vi "Pulse convert.vi"(11 "PulseIN":i32) -> (2 "Speed(rpm)":i16, 3 "Speed(rad/s)":dbl)   [LabVIEW 2019]
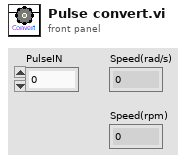
[diagram p1: front panel]
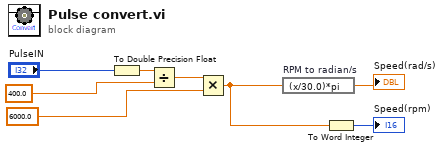
[diagram p0: block diagram]
diagram:
  n1 = To Double Precision Float(number="PulseIN") -> (double precision float=w1:dbl)
  n2 = Divide(x=w1, y=400.0) -> (x/y=w3:dbl)
  n3 = Multiply(x=w3, y=6000.0) -> (x*y=w5:dbl)
  n4 = expression code="(x/30.0)*pi" "RPM to radian/s"(w5) -> (→"Speed(rad/s)":dbl)
  n5 = To Word Integer(number=w5) -> (16bit integer=→"Speed(rpm)":i16)
